vi "GetTargetDepthColumnIndex.vi"(11 "Tab Array":string[][](array[string])) -> (2 "Found?":bool, 3 "Start Index":i32)   [LabVIEW 2012]
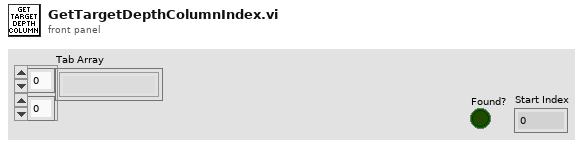
[diagram p1: front panel]
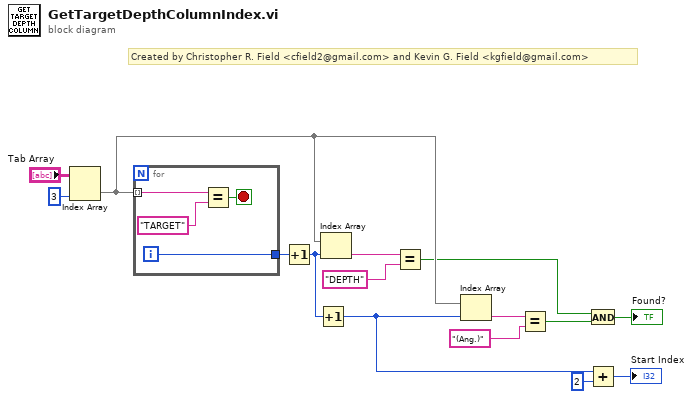
[diagram p0: block diagram]
diagram:
  # "Created by Christopher R. Field <cfield2@gmail.com> and Kevin G. Field <kgfield@gmail.com>"
  n1 = Index Array(array="Tab Array", index (col)=3 ("disabled index (col)")) -> (element=w9:string[])  [unwired: 1 in]
  n2 = for {
    tunnel: w9 -> [w19] mode=indexing
    tunnel: [w16] -> w13
    i -> [w16]
    stop <- w17 stop-if-true
    n3 = Equal?(x=w19, y="TARGET") -> (x = y?=w17:bool)
  }
  n4 = Increment(x=w13) -> (x+1=w10:i32)
  n5 = Increment(x=w10) -> (x+1=w6:i32)
  n6 = Index Array(array=w9, index=w10) -> (element=w12:string)
  n7 = Equal?(x=w12, y="DEPTH") -> (x = y?=w4:bool)
  n8 = Index Array(array=w9, index=w6) -> (element=w8:string)
  n9 = Equal?(x=w8, y="(Ang.)") -> (x = y?=w3:bool)
  n10 = And(x=w4, y=w3) -> (x .and. y?=→"Found?":bool)
  n11 = Add(x=w6, y=2) -> (x+y=→"Start Index":i32)
